vi "Agilent ESG Series Config NADC Signal.vi"() -> ()   [LabVIEW 2012]
doc: "This application VI for the Hewlett Packard ESG/ESG-D Series Signal Generator will open a VISA session and configure the signal generator to output a pi/4DQPSK digitally-modulated signal in a NADC format with the following characteristics:\nCarrier frequency set to 835 MHz\nPower level set to 0 dBm\nTimeslot 1 activated and configured as an Uplink Custom channel\nA fixed 4-bit repeating sequence as an uplink Traffic channel\nTimeslot 3 activated and configured as an Uplink Traffic channel\nA repeating pattern of 4 1's and 4 0's selected as the data pattern for timeslot 3.\n\nIt will then check for errors and close the session.\n\nNotes:\nThe VI is available for ESG-A and ESG-D Series instruments only because of Config Frequency.vi."
uses:
  Agilent ESG Series.lvlib
panel:
  in  "Timeslot 3 Type (2:UP TCH)":T1(ring)=enum."UP TCH"
  in  "Timeslot 1 Type (0:UP CUSTOM)":T1(ring)
  in  "Timeslot 3 FIX4 (0000)":i16 format="%.0b"
  in  "Timeslot 1 FIX4 (1010)":i16=10 format="%.0b"
  in  "Timeslot 3 Data (5:4 1's&4 0's)":T2(ring)=enum."4 1's & 4 0's"
  in  "Timeslot 1 Data (0:PN9)":T2(ring)=enum."FIX4"
  in  "Unit (0:dBm)":T3(ring)
  in  "Amplitude (0.0)":dbl format="%.2f"
  in  "Frequency (835.0)":dbl=835.0 format="%.5f"
  in  "error in (no error)":errorcluster {"code" format="%.0x"}
  out "error out":errorcluster {"code" format="%.0x"}
  in  "VISA session":refnum<visa-resource-name>
  # "(c) 2005 - 2013 National Instruments.  ALL RIGHTS RESERVED."
  # "ESG/ESG-D"
  # "Series Signal Generator"
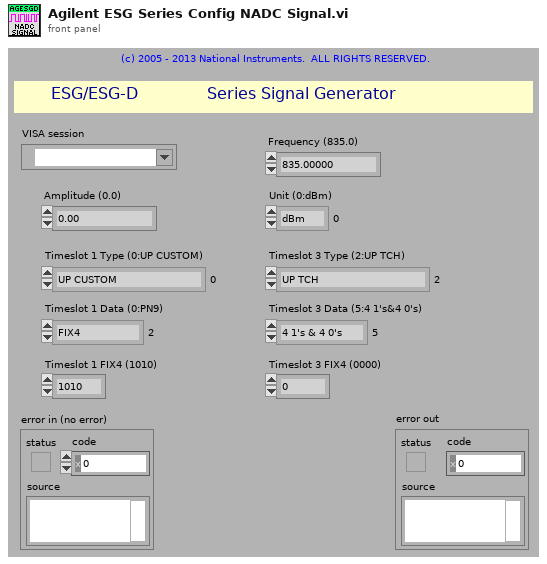
[diagram p1: front panel]
types:
  T1 = enum16{"UP CUSTOM", "DOWN CUSTOM", "UP TCH", "DOWN TCH", "UP TCH ALL", "DOWN TCH ALL"}
  T2 = enum16{"PN9", "PN15", "FIX4", "USER FILE", "EXT", "4 1's & 4 0's", "8 1's & 8 0's", "16 1's & 16 0's", "32 1's & 32 0's", "64 1's & 64 0's"}
  T3 = enum16{"dBm", "dBuV", "dBuVemf", "mV", "uV", "mVemf", "uVemf"}
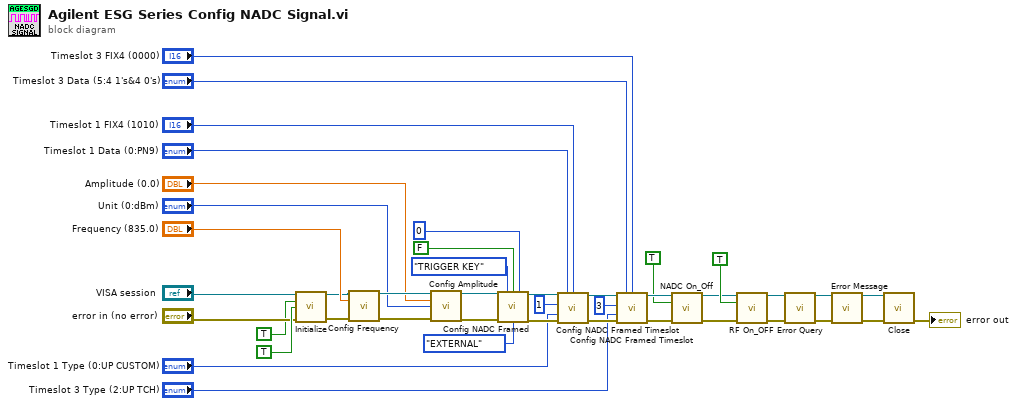
[diagram p0: block diagram]
diagram:
  n1 = call "Initialize.vi"("VISA Resource Name"="VISA session", "ID Query? (T: Yes)"=TRUE, "Reset? (T: Yes)"=TRUE, "error in (no error)"="error in (no error)") -> ("VISA Resource Name Out"=w16:refnum<visa-resource-name>, "error out"=w15:errorcluster)  [unwired: 10 in]
  n2 = call "Config Frequency.vi"("VISA Resource Name"=w16, "Frequency (1000.0)"="Frequency (835.0)", "error in (no error)"=w15) -> ("VISA Resource Name Out"=w42:refnum<visa-resource-name>, "error out"=w41:errorcluster)  [unwired: 11 in]
  n3 = call "Config Amplitude.vi"("VISA Resource Name"=w42, "Amplitude (-135.00)"="Amplitude (0.0)", "Unit (0:dBm)"="Unit (0:dBm)", "error in (no error)"=w41) -> ("VISA Resource Name Out"=w40:refnum<visa-resource-name>, "error out"=w34:errorcluster)  [unwired: 10 in]
  n4 = call "Config NADC Framed.vi"("VISA Resource Name"=w40, "Frame Trigger (2:TRIGGER KEY)"=enum16{"BUS", "EXTERNAL", "TRIGGER KEY"}."TRIGGER KEY", "Ext Delay (F:OFF)"=FALSE, "Ext Delay Bits (0)"=0, "error in (no error)"=w34, "Sec Frame Trigger (1:EXT)"=enum16{"BUS", "EXTERNAL", "TRIGGER KEY"}."EXTERNAL") -> ("VISA Resource Name Out"=w33:refnum<visa-resource-name>, "error out"=w32:errorcluster)  [unwired: 8 in]
  n5 = call "Config NADC Framed Timeslot.vi"("VISA Resource Name"=w33, "Data (0:PN9)"="Timeslot 1 Data (0:PN9)", "FIX4 (0000)"="Timeslot 1 FIX4 (1010)", "Timeslot (1)"=i16 1, "Timeslot Type (2:UP TCH)"="Timeslot 1 Type (0:UP CUSTOM)", "error in (no error)"=w32) -> ("VISA Resource Name Out"=w30:refnum<visa-resource-name>, "error out"=w31:errorcluster)  [unwired: 8 in]
  n6 = call "Config NADC Framed Timeslot.vi"("VISA Resource Name"=w30, "Data (0:PN9)"="Timeslot 3 Data (5:4 1's&4 0's)", "FIX4 (0000)"="Timeslot 3 FIX4 (0000)", "Timeslot (1)"=i16 3, "Timeslot Type (2:UP TCH)"="Timeslot 3 Type (2:UP TCH)", "error in (no error)"=w31) -> ("VISA Resource Name Out"=w27:refnum<visa-resource-name>, "error out"=w26:errorcluster)  [unwired: 8 in]
  n7 = call "NADC On_Off.vi"("VISA Resource Name"=w27, "NADC (T:ON)"=TRUE, "error in (no error)"=w26) -> ("VISA Resource Name Out"=w24:refnum<visa-resource-name>, "error out"=w25:errorcluster)  [unwired: 11 in]
  n8 = call "RF On_OFF.vi"("VISA Resource Name"=w24, "Status (T:ON)"=TRUE, "error in (no error)"=w25) -> ("VISA Resource Name Out"=w5:refnum<visa-resource-name>, "error out"=w6:errorcluster)  [unwired: 11 in]
  n9 = call "Error Query.vi"("VISA Resource Name"=w5, "error in (no error)"=w6) -> ("VISA Resource Name Out"=w8:refnum<visa-resource-name>, "error out"=w7:errorcluster)  [unwired: 10 in, 2 out]
  n10 = call "Error Message.vi"("VISA Resource Name"=w8, "error in (no error)"=w7) -> ("VISA Resource Name Out"=w9:refnum<visa-resource-name>, "error out"=w10:errorcluster)  [unwired: 9 in, 3 out]
  n11 = call "Close.vi"("VISA Resource Name"=w9, "error in (no error)"=w10) -> ("error out"=→"error out":errorcluster)  [unwired: 13 in]
